vi "Send PCP command.vi"(0 "PSU type":T1, 1 "PCP":T2, 7 "SP":dbl, 11 "error out 2":errorcluster) -> (6 "d(0.0)":dbl, 8 "Final motor voltage update made":bool, 10 "Updated motor voltage pending":bool, 15 "error out":errorcluster)   [LabVIEW 2011]
uses:
  High Level/PCP High Level Commands.ctl
  PSU Type.ctl
  PCP Commands.ctl
  PCP Command definer.ctl
  Magna Interface/Magna Commands.ctl
  Magna Interface/Magna Command Definer.ctl
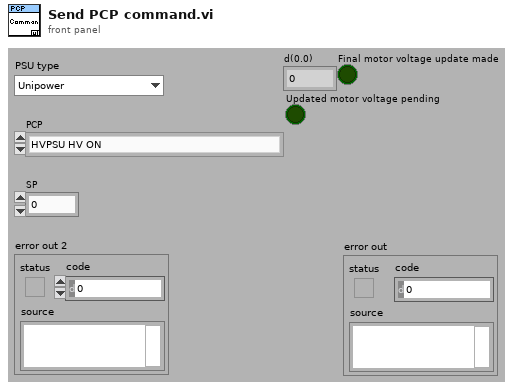
[diagram p1: front panel]
types:
  T1 = typedef "PSU Type.ctl" = enum16{"Unipower", "Magna 8.3A", "Magna 12A", "None"}
  T2 = typedef "PCP High Level Commands.ctl" = enum16{"HVPSU HV ON", "HVPSU HV OFF", "PCP PC", "PCP Local", "Update Motor Voltage", "Update Cable Resistance", "Final Motor Voltage", "Final Resistance"}
  T3 = typedef "PCP Commands.ctl" = enum16{"do not use HE - Help", "RDd - Most used inputs", "RA - All analog inputs", "RE n Reset DO n", "SE n Set DO n", "RP - Get digital inputs", "VA d Set AO A  Motor Volt", "VB d Set AO B  Cable Resistance", "VEr - Get Version", "DYp - Depth counter", "DR - Reset Depth Counter", "DS n Set Depth options(0-3)", "do not use ME - Manual mode enabled", "MD - Manual mode disabled", "ID - Get ID(2001)", "TS - Get Timestamp", "TO d(s)  Set timeout", "do not use LO n Start Loop Mode(1,2)", "AL n RD&LO variation", "ST - Stop Loop Mode"}
  T4 = typedef "PCP Command definer.ctl" = cluster{"Action":T3, "n(0)":i32, "d(0.0)":dbl}
  T5 = typedef "Magna Commands.ctl" = enum16{"Read Inputs", "HV ON", "HV OFF", "Set Resistance", "Set Head Voltage SP"}
  T6 = typedef "Magna Command Definer.ctl" = cluster{"Action":T5, "n(0)":i32, "d(0.0)":dbl}
  T7 = typedef "Options  All pages and custom.ctl" = cluster{"P 1 (App)":T8, "P 2":T9, "P 3":T10, "P 4":T12, "P 5":T17, "P 6 (Err)":T18, "P 7 (Expert)":T19, "P 8 (Depth)":T21, "C 1":T22, "C 2":T23}
  T8 = typedef "Options Page 1 (App).ctl" = cluster{"Result files":path, "PCP Interface":string, "Tractor/Stroker Interface":string, "Tractor Interface":string, "Modem Status Interface":string, "Audible Alarm":bool, "Force alarm on Technical":bool, "Force alarm on HH":bool, "Force alarm on LL":bool, "Force alarm on H":bool, "Force alarm on L":bool}
  T9 = typedef "Options Page 2.ctl" = cluster{"Solenoid & Relay latching time":u16, "Tractor relay 1":dbl, "Tractor relay 2":dbl, "Tractor Solenoid limit":dbl}
  T10 = typedef "Options Page 3.ctl" = cluster{"Min resistance":dbl, "Max resistance":dbl, "Head voltage range":T11, "Max voltage jump":dbl, "Maximum resistance change":dbl, "Start Telemetry Voltage":dbl, "Start Telemetry Timeout":dbl, "Start Motor Voltage":dbl, "Stop Motor Voltage":dbl, "Pass Mode Warning Voltage":dbl, "Relay Switch Voltage":dbl, "Relay Status Loss Voltage":dbl, "Samples to average":i32, "PSU type DO NOT USE":T1, "Magna OVP":dbl, "Magna Current Limit":dbl}
  T11 = typedef "PCP type List.ctl" = enum16{"0 - 350V", "0 - 450V", "0 - 600V"}
  T12 = typedef "Options Page 4.ctl" = cluster{"Solenoid & Relay latching time":u16, "Stroker relay 1":dbl, "Stroker Relay 2":dbl, "Stroker Solenoid limit":dbl, "Force det.":T13, "Stroke force lim.":dbl, "Anchor Enabled Pressure":dbl, "Tacometer puls":dbl, "Default anchor behavior":T14, "Default stroker behavior":T15, "Default stroker force limit (tonne)":dbl, "Slips Size":T16}
  T13 = typedef "Stroke force selector.ctl" = enum16{"Stroke in = node 1", "Strok out = node 1"}
  T14 = typedef "Default anchor behavior.ctl" = enum16{"Do nothing", "Set Anchor", "Release Anchor"}
  T15 = typedef "Default stroker behavior.ctl" = enum16{"Do nothing", "Stop", "Go Out", "Go In"}
  T16 = typedef "Slips Type Radio.ctl" = enum32{"No Selection", "338 MRS", "3,9 MRS"}
  T17 = typedef "Options Page 5.ctl" = cluster{"Solenoid & Relay latching time":u16, "Driller relay 1":dbl, "Driller Relay 2":dbl, "Driller  Solenoid limit":dbl}
  T18 = typedef "Options Page 6 (Err).ctl" = cluster{"Error and event files":path}
  T19 = typedef "Options Page 7 (Expert).ctl" = cluster{"Show Debug":bool, "Log debug messages":bool, "Additional debug messages":bool, "Start Beagle with Simulator data":bool, "Workshop mode":bool, "Modem baud":u16, "enumCANCOM":bool, "Modem sim":T20, "Telemetry Timeout Disable":i32, "Buffer size":i32, "Upd regular data":bool, "Cable comp":cluster{"VMOD1 Voltage(V)":dbl, "VMOD2 Voltage(V)":dbl}}
  T20 = typedef "Modem simulation setup.ctl" = cluster{"Modem dealay sim":bool, "Sim baud Tx":u16, "Bit Error fraction Tx":dbl, "Sim baud Rx":u16, "Bit Error fraction Rx":dbl}
  T21 = typedef "Options Page 8 (Depth).ctl" = cluster{"Winch Spool Circumference":dbl, "Winch Pulses per Revolution":dbl, "Current Depth":dbl}
  T22 = typedef "Options Custom 1.ctl" = cluster{"Depth Updated":bool, "Depth Offset":dbl}
  T23 = typedef "Options Custom 2.ctl" = cluster{"Placeholder":bool}
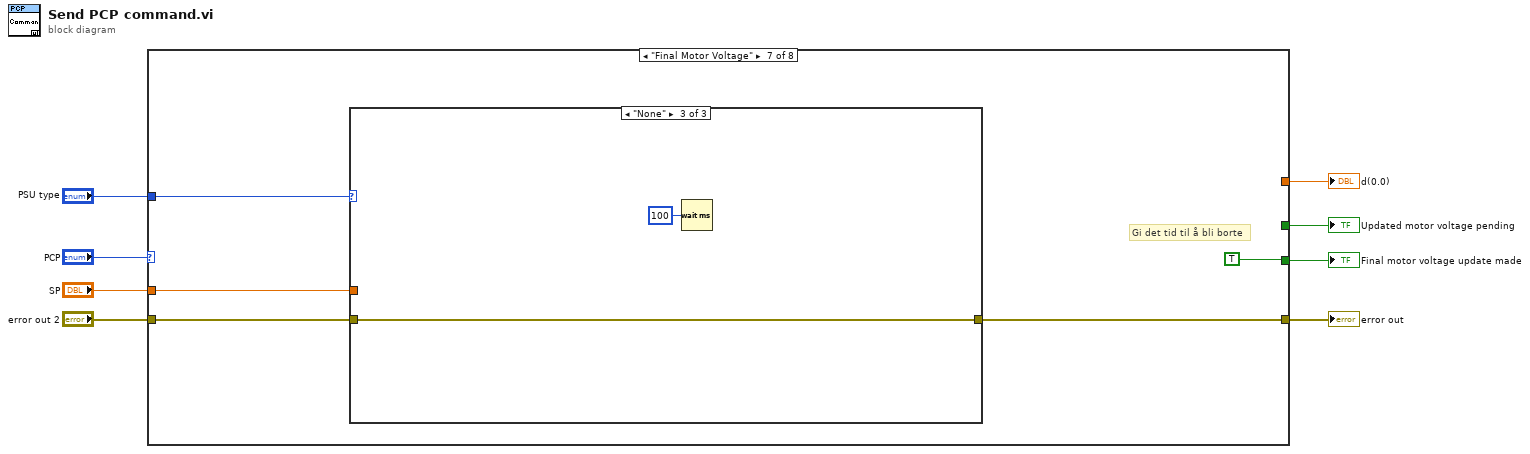
[diagram p0: block diagram]
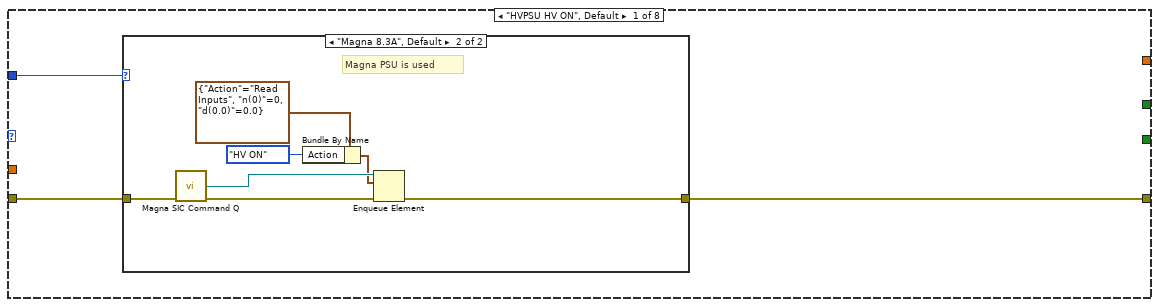
[diagram p2: hidden frame]
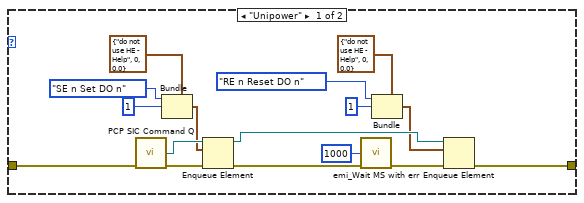
[diagram p3: hidden frame]
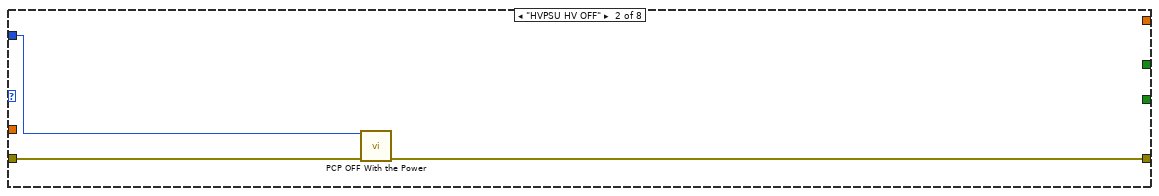
[diagram p4: hidden frame]
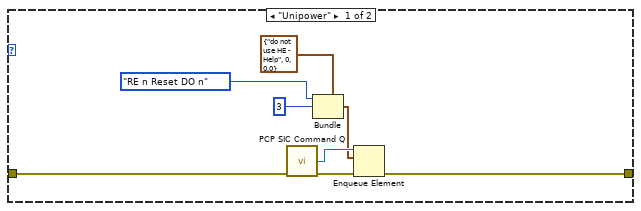
[diagram p6: hidden frame]
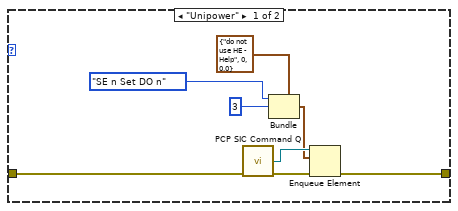
[diagram p8: hidden frame]
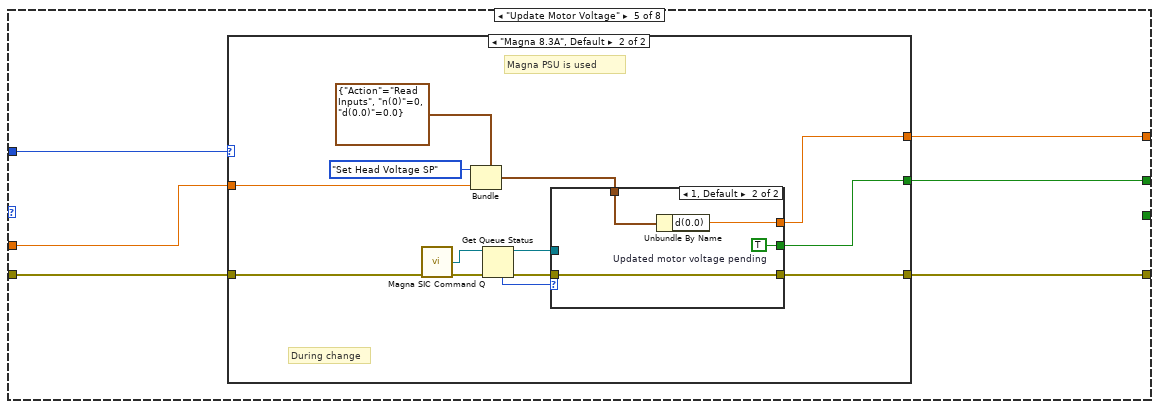
[diagram p9: hidden frame]
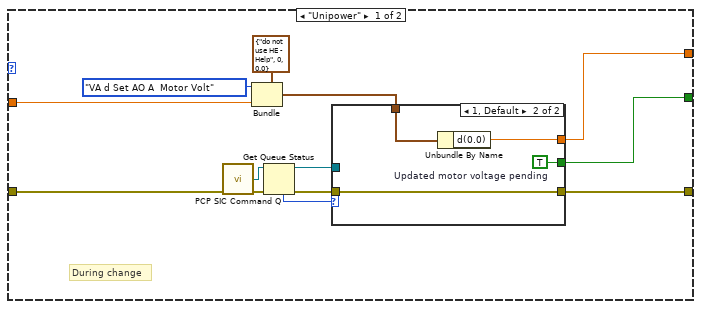
[diagram p10: hidden frame]
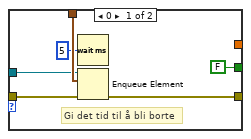
[diagram p11: hidden frame]
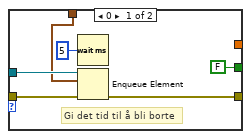
[diagram p12: hidden frame]
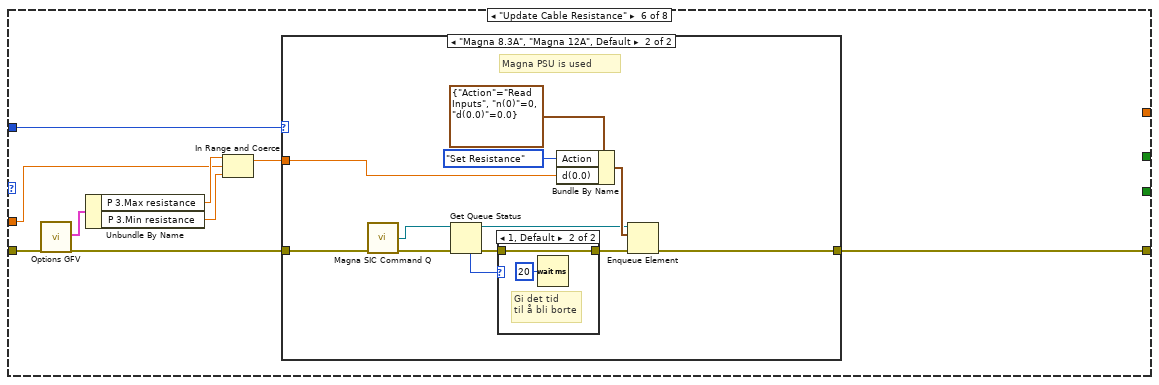
[diagram p13: hidden frame]
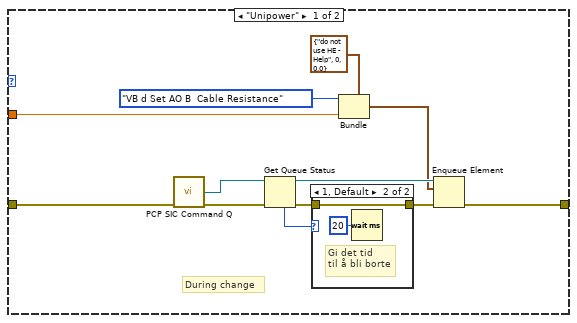
[diagram p14: hidden frame]
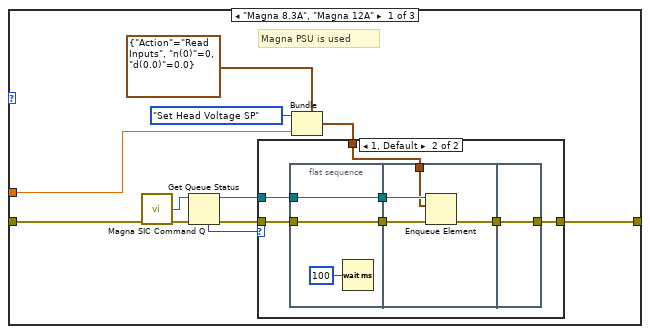
[diagram p17: hidden frame]
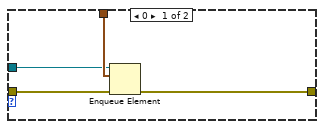
[diagram p18: hidden frame]
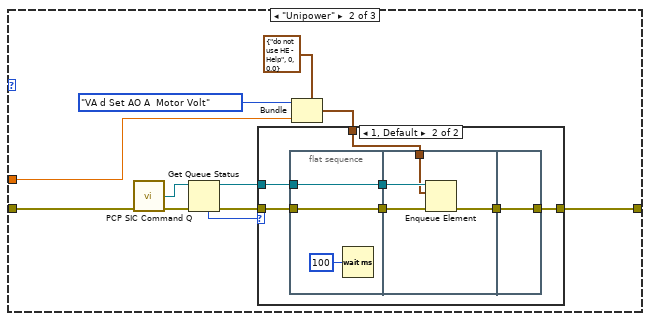
[diagram p19: hidden frame]
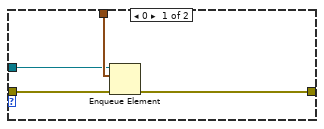
[diagram p20: hidden frame]
diagram:
  n1 = case shown="\"Final Motor Voltage\"" "PCP" {
    tunnel: "error out 2" -> [w11 w36 w40 w52 w67 w119 w157 w226]
    tunnel: "SP" -> [_ _ _ _ w66 w118 w156 w222]
    tunnel: [w10 w37 w39 w51 w65 w115 w155 w228] -> w8
    tunnel: [_ _ _ _ w64 _ _ _] -> w4
    tunnel: [_ _ _ _ w63 _ _ _] -> w3
    tunnel: [_ _ _ _ _ _ TRUE _] -> w2
    tunnel: "PSU type" -> [w9 w35 w38 w50 w62 w114 w153 w220]
    frame "HVPSU HV ON", Default {
      n2 = case shown="\"Magna 8.3A\", Default" w9 {
        tunnel: w11 -> [w13 w34]
        tunnel: [w12 w28] -> w10
        frame "Unipower" {
          n3 = call "PCP SIC Command Q.vi"("error in (no error)"=w13) -> ("PCP cmd Q"=w26:refnum<queue>, "error out"=w27:errorcluster)  [unwired: 13 in]
          n4 = Bundle(cluster=T4 {"Action"=enum."do not use HE - Help", "n(0)"=0, "d(0.0)"=0.0} ("PCP command definer"), "Action"=PCP_Commands."SE n Set DO n", "n(0)"=1) -> (w20:T4)  [unwired: 1 in]
          n5 = Enqueue Element(queue=w26, element=w20, error in (no error)=w27) -> (queue out=w22:refnum<queue>, error out=w25:errorcluster)  [unwired: 1 in, 1 out]
          n6 = call "emi_Wait MS with err.vi"("milliseconds to wait(0)"=u32 1000, "error in (no error)"=w25) -> ("error out"=w23:errorcluster)  [unwired: 13 in]
          n7 = Bundle(cluster=T4 {"Action"=enum."do not use HE - Help", "n(0)"=0, "d(0.0)"=0.0} ("PCP command definer"), "Action"=PCP_Commands."RE n Reset DO n", "n(0)"=1) -> (w18:T4)  [unwired: 1 in]
          n8 = Enqueue Element(queue=w22, element=w18, error in (no error)=w23) -> (error out=w12:errorcluster)  [unwired: 1 in, 2 out]
        }
        frame "Magna 8.3A", Default {
          # "Magna PSU is used"
          n9 = call "Magna SIC Command Q.vi"("error in (no error)"=w34) -> ("queue out"=w32:refnum<queue>, "error out"=w33:errorcluster)  [unwired: 13 in]
          n10 = Bundle By Name(cluster=T6 {"Action"=enum."Read Inputs", "n(0)"=0, "d(0.0)"=0.0} ("element"), "Action"=Magna_Commands."HV ON") -> (w30:T6)
          n11 = Enqueue Element(queue=w32, element=w30, error in (no error)=w33) -> (error out=w28:errorcluster)  [unwired: 1 in, 2 out]
        }
      }
    }
    frame "HVPSU HV OFF" {
      n12 = call "PCP OFF With the Power.vi"("PSU type"=w35, "error In"=w36) -> ("error out"=w37:errorcluster)  [unwired: 13 in]
    }
    frame "PCP PC" {
      n13 = case shown="\"Magna 8.3A\", Default" w38 {
        tunnel: w40 -> [w48 w49]
        tunnel: [w41 w49] -> w39
        frame "Unipower" {
          n14 = call "PCP SIC Command Q.vi"("error in (no error)"=w48) -> ("PCP cmd Q"=w46:refnum<queue>, "error out"=w47:errorcluster)  [unwired: 13 in]
          n15 = Bundle(cluster=T4 {"Action"=enum."do not use HE - Help", "n(0)"=0, "d(0.0)"=0.0} ("PCP command definer"), "Action"=PCP_Commands."RE n Reset DO n", "n(0)"=3) -> (w44:T4)  [unwired: 1 in]
          n16 = Enqueue Element(queue=w46, element=w44, error in (no error)=w47) -> (error out=w41:errorcluster)  [unwired: 1 in, 2 out]
        }
        frame "Magna 8.3A", Default {
          # "Command is not supported"
          # "Magna PSU is used"
        }
      }
    }
    frame "PCP Local" {
      n17 = case shown="\"Magna 8.3A\", Default" w50 {
        tunnel: w52 -> [w60 w61]
        tunnel: [w53 w61] -> w51
        frame "Unipower" {
          n18 = call "PCP SIC Command Q.vi"("error in (no error)"=w60) -> ("PCP cmd Q"=w58:refnum<queue>, "error out"=w59:errorcluster)  [unwired: 13 in]
          n19 = Bundle(cluster=T4 {"Action"=enum."do not use HE - Help", "n(0)"=0, "d(0.0)"=0.0} ("PCP command definer"), "Action"=PCP_Commands."SE n Set DO n", "n(0)"=3) -> (w56:T4)  [unwired: 1 in]
          n20 = Enqueue Element(queue=w58, element=w56, error in (no error)=w59) -> (error out=w53:errorcluster)  [unwired: 1 in, 2 out]
        }
        frame "Magna 8.3A", Default {
          # "Command is not supported"
          # "Magna PSU is used"
        }
      }
    }
    frame "Update Motor Voltage" {
      n21 = case shown="\"Magna 8.3A\", Default" w62 {
        tunnel: w67 -> [w77 w95]
        tunnel: w66 -> [w76 w102]
        tunnel: [w71 w99] -> w65
        tunnel: [w69 w97] -> w64
        tunnel: [w68 w96] -> w63
        frame "Unipower" {
          # "During change"
          n22 = call "PCP SIC Command Q.vi"("error in (no error)"=w77) -> ("PCP cmd Q"=w74:refnum<queue>, "error out"=w75:errorcluster)  [unwired: 13 in]
          n23 = Bundle(cluster=T4 {"Action"=enum."do not use HE - Help", "n(0)"=0, "d(0.0)"=0.0} ("PCP command definer"), "Action"=PCP_Commands."VA d Set AO A  Motor Volt", "d(0.0)"=w76) -> (w79:T4)  [unwired: 1 in]
          n24 = Get Queue Status(queue=w74, error in (no error)=w75) -> (queue out=w70:refnum<queue>, error out=w73:errorcluster, # elements in queue=w72:i32)  [unwired: 1 in, 5 out]
          n25 = case shown="1, Default" w72 {
            tunnel: w79 -> [w86 w89]
            tunnel: w73 -> [w85 w90]
            tunnel: [w84 w90] -> w71
            tunnel: w70 -> [w83 _]
            tunnel: [_ w88] -> w69
            tunnel: [FALSE ("Updated motor voltage pending") w87] -> w68
            frame 0 {
              # "Gi det tid til å bli borte"
              n26 = Wait (ms)(milliseconds to wait=u32 5) -> ()  [unwired: 1 out]
              n27 = Enqueue Element(queue=w83, element=w86, error in (no error)=w85) -> (error out=w84:errorcluster)  [unwired: 1 in, 2 out]
            }
            frame 1, Default {
              w87 = TRUE  # Updated motor voltage pending
              n28 = Unbundle By Name(w89) -> ("d(0.0)"=w88:dbl)
            }
          }
        }
        frame "Magna 8.3A", Default {
          # "Magna PSU is used"
          # "During change"
          n29 = call "Magna SIC Command Q.vi"("error in (no error)"=w95) -> ("queue out"=w93:refnum<queue>, "error out"=w94:errorcluster)  [unwired: 13 in]
          n30 = Bundle(cluster=T6 {"Action"=enum."Read Inputs", "n(0)"=0, "d(0.0)"=0.0} ("element"), "Action"=Magna_Commands."Set Head Voltage SP", "d(0.0)"=w102) -> (w103:T6)  [unwired: 1 in]
          n31 = Get Queue Status(queue=w93, error in (no error)=w94) -> (queue out=w98:refnum<queue>, error out=w101:errorcluster, # elements in queue=w100:i32)  [unwired: 1 in, 5 out]
          n32 = case shown="1, Default" w100 {
            tunnel: w103 -> [w104 w112]
            tunnel: w101 -> [w109 w113]
            tunnel: [w108 w113] -> w99
            tunnel: w98 -> [w107 _]
            tunnel: [_ w111] -> w97
            tunnel: [FALSE ("Updated motor voltage pending") w110] -> w96
            frame 0 {
              # "Gi det tid til å bli borte"
              n33 = Wait (ms)(milliseconds to wait=u32 5) -> ()  [unwired: 1 out]
              n34 = Enqueue Element(queue=w107, element=w104, error in (no error)=w109) -> (error out=w108:errorcluster)  [unwired: 1 in, 2 out]
            }
            frame 1, Default {
              w110 = TRUE  # Updated motor voltage pending
              n35 = Unbundle By Name(w112) -> ("d(0.0)"=w111:dbl)
            }
          }
        }
      }
    }
    frame "Update Cable Resistance" {
      n36 = call "Options GFV.vi"("error in (no error)"=w119) -> ("Options"=w122:T7, "error out"=w116:errorcluster)  [unwired: 16 in, 1 out]
      n37 = Unbundle By Name(w122) -> ("P 3.Max resistance"=w121:dbl, "P 3.Min resistance"=w120:dbl)
      n38 = In Range and Coerce(upper limit=w121, x=w118, lower limit=w120) -> (coerced(x)=w117:dbl)  [unwired: 1 out]
      n39 = case shown="\"Magna 8.3A\", \"Magna 12A\", Default" w114 {
        tunnel: w117 -> [w132 w138]
        tunnel: w116 -> [w125 w146]
        tunnel: [w124 w145] -> w115
        frame "Unipower" {
          # "During change"
          n40 = call "PCP SIC Command Q.vi"("error in (no error)"=w125) -> ("PCP cmd Q"=w126:refnum<queue>, "error out"=w127:errorcluster)  [unwired: 13 in]
          n41 = Get Queue Status(queue=w126, error in (no error)=w127) -> (queue out=w128:refnum<queue>, error out=w131:errorcluster, # elements in queue=w130:i32)  [unwired: 1 in, 5 out]
          n42 = case shown="1, Default" w130 {
            tunnel: w131 -> [w135 w136]
            tunnel: [w135 w136] -> w129
            frame 0 {
            }
            frame 1, Default {
              # "Gi det tid \ntil å bli borte"
              n43 = Wait (ms)(milliseconds to wait=u32 20) -> ()  [unwired: 1 out]
            }
          }
          n44 = Bundle(cluster=T4 {"Action"=enum."do not use HE - Help", "n(0)"=0, "d(0.0)"=0.0} ("PCP command definer"), "Action"=PCP_Commands."VB d Set AO B  Cable Resistance", "d(0.0)"=w132) -> (w123:T4)  [unwired: 1 in]
          n45 = Enqueue Element(queue=w128, element=w123, error in (no error)=w129) -> (error out=w124:errorcluster)  [unwired: 1 in, 2 out]
        }
        frame "Magna 8.3A", "Magna 12A", Default {
          # "Magna PSU is used"
          n46 = call "Magna SIC Command Q.vi"("error in (no error)"=w146) -> ("queue out"=w141:refnum<queue>, "error out"=w142:errorcluster)  [unwired: 13 in]
          n47 = Get Queue Status(queue=w141, error in (no error)=w142) -> (queue out=w140:refnum<queue>, error out=w144:errorcluster, # elements in queue=w143:i32)  [unwired: 1 in, 5 out]
          n48 = case shown="1, Default" w143 {
            tunnel: w144 -> [w150 w151]
            tunnel: [w150 w151] -> w139
            frame 0 {
            }
            frame 1, Default {
              # "Gi det tid \ntil å bli borte"
              n49 = Wait (ms)(milliseconds to wait=u32 20) -> ()  [unwired: 1 out]
            }
          }
          n50 = Bundle By Name(cluster=T6 {"Action"=enum."Read Inputs", "n(0)"=0, "d(0.0)"=0.0} ("element"), "Action"=Magna_Commands."Set Resistance", "d(0.0)"=w138) -> (w148:T6)
          n51 = Enqueue Element(queue=w140, element=w148, error in (no error)=w139) -> (error out=w145:errorcluster)  [unwired: 1 in, 2 out]
        }
      }
    }
    frame "Final Motor Voltage" {
      # "Gi det tid til å bli borte"
      n52 = case shown="\"None\"" w153 {
        tunnel: w157 -> [w160 w195 w218]
        tunnel: w156 -> [w167 w194 _]
        tunnel: [w164 w189 w218] -> w155
        frame "Magna 8.3A", "Magna 12A" {
          # "Magna PSU is used"
          n53 = call "Magna SIC Command Q.vi"("error in (no error)"=w160) -> ("queue out"=w158:refnum<queue>, "error out"=w159:errorcluster)  [unwired: 13 in]
          n54 = Get Queue Status(queue=w158, error in (no error)=w159) -> (queue out=w163:refnum<queue>, error out=w166:errorcluster, # elements in queue=w165:i32)  [unwired: 1 in, 5 out]
          n55 = Bundle(cluster=T6 {"Action"=enum."Read Inputs", "n(0)"=0, "d(0.0)"=0.0} ("element"), "Action"=Magna_Commands."Set Head Voltage SP", "d(0.0)"=w167) -> (w168:T6)  [unwired: 1 in]
          n56 = case shown="1, Default" w165 {
            tunnel: w168 -> [w172 w176]
            tunnel: w166 -> [w171 w179]
            tunnel: [w170 w174] -> w164
            tunnel: w163 -> [w169 w177]
            frame 0 {
              n57 = Enqueue Element(queue=w169, element=w172, error in (no error)=w171) -> (error out=w170:errorcluster)  [unwired: 1 in, 2 out]
            }
            frame 1, Default {
              n58 = flat-sequence {
                tunnel: w179 -> [w180]
                tunnel: [w181] -> w178
                tunnel: w177 -> [w181]
                tunnel: [w180] -> w175
                tunnel: w178 -> [w186]
                tunnel: w176 -> [w185]
                tunnel: w175 -> [w184]
                tunnel: [w183] -> w173
                tunnel: [w187] -> w174
                tunnel: w173 -> [w187]
                frame #0 {
                  n59 = Wait (ms)(milliseconds to wait=u32 100) -> ()  [unwired: 1 out]
                }
                frame #1 {
                  n60 = Enqueue Element(queue=w186, element=w185, error in (no error)=w184) -> (error out=w183:errorcluster)  [unwired: 1 in, 2 out]
                }
                frame #2 {
                }
              }
            }
          }
        }
        frame "Unipower" {
          n61 = call "PCP SIC Command Q.vi"("error in (no error)"=w195) -> ("PCP cmd Q"=w192:refnum<queue>, "error out"=w193:errorcluster)  [unwired: 13 in]
          n62 = Get Queue Status(queue=w192, error in (no error)=w193) -> (queue out=w188:refnum<queue>, error out=w191:errorcluster, # elements in queue=w190:i32)  [unwired: 1 in, 5 out]
          n63 = Bundle(cluster=T4 {"Action"=enum."do not use HE - Help", "n(0)"=0, "d(0.0)"=0.0} ("PCP command definer"), "Action"=PCP_Commands."VA d Set AO A  Motor Volt", "d(0.0)"=w194) -> (w197:T4)  [unwired: 1 in]
          n64 = case shown="1, Default" w190 {
            tunnel: w197 -> [w202 w206]
            tunnel: w191 -> [w201 w209]
            tunnel: [w200 w204] -> w189
            tunnel: w188 -> [w199 w207]
            frame 0 {
              n65 = Enqueue Element(queue=w199, element=w202, error in (no error)=w201) -> (error out=w200:errorcluster)  [unwired: 1 in, 2 out]
            }
            frame 1, Default {
              n66 = flat-sequence {
                tunnel: w209 -> [w210]
                tunnel: [w211] -> w208
                tunnel: w207 -> [w211]
                tunnel: [w210] -> w205
                tunnel: w208 -> [w216]
                tunnel: w206 -> [w215]
                tunnel: w205 -> [w214]
                tunnel: [w213] -> w203
                tunnel: [w217] -> w204
                tunnel: w203 -> [w217]
                frame #0 {
                  n67 = Wait (ms)(milliseconds to wait=u32 100) -> ()  [unwired: 1 out]
                }
                frame #1 {
                  n68 = Enqueue Element(queue=w216, element=w215, error in (no error)=w214) -> (error out=w213:errorcluster)  [unwired: 1 in, 2 out]
                }
                frame #2 {
                }
              }
            }
          }
        }
        frame "None" {
          n69 = Wait (ms)(milliseconds to wait=u32 100) -> ()  [unwired: 1 out]
        }
      }
    }
    frame "Final Resistance" {
      n70 = call "Options GFV.vi"("error in (no error)"=w226) -> ("Options"=w227:T7, "error out"=w225:errorcluster)  [unwired: 16 in, 1 out]
      n71 = Unbundle By Name(w227) -> ("P 3.Max resistance"=w224:dbl, "P 3.Min resistance"=w223:dbl)
      n72 = In Range and Coerce(upper limit=w224, x=w222, lower limit=w223) -> (coerced(x)=w221:dbl)  [unwired: 1 out]
      n73 = case shown="\"Magna 8.3A\", Default" w220 {
        tunnel: [w229 w244] -> w228
        tunnel: w225 -> [w238 w250]
        tunnel: w221 -> [w237 w253]
        frame "Unipower" {
          n74 = call "PCP SIC Command Q.vi"("error in (no error)"=w238) -> ("PCP cmd Q"=w231:refnum<queue>, "error out"=w232:errorcluster)  [unwired: 13 in]
          n75 = Get Queue Status(queue=w231, error in (no error)=w232) -> (queue out=w233:refnum<queue>, error out=w236:errorcluster, # elements in queue=w235:i32)  [unwired: 1 in, 5 out]
          n76 = case shown="1, Default" w235 {
            tunnel: w236 -> [w241 w242]
            tunnel: [w241 w242] -> w234
            frame 0 {
            }
            frame 1, Default {
              # "Gi det tid \ntil å bli borte"
              n77 = Wait (ms)(milliseconds to wait=u32 100) -> ()  [unwired: 1 out]
            }
          }
          n78 = Bundle(cluster=T4 {"Action"=enum."do not use HE - Help", "n(0)"=0, "d(0.0)"=0.0} ("PCP command definer"), "Action"=PCP_Commands."VB d Set AO B  Cable Resistance", "d(0.0)"=w237) -> (w230:T4)  [unwired: 1 in]
          n79 = Enqueue Element(queue=w233, element=w230, error in (no error)=w234) -> (error out=w229:errorcluster)  [unwired: 1 in, 2 out]
        }
        frame "Magna 8.3A", Default {
          # "Magna PSU is used"
          n80 = call "Magna SIC Command Q.vi"("error in (no error)"=w250) -> ("queue out"=w251:refnum<queue>, "error out"=w252:errorcluster)  [unwired: 13 in]
          n81 = Get Queue Status(queue=w251, error in (no error)=w252) -> (queue out=w245:refnum<queue>, error out=w255:errorcluster, # elements in queue=w254:i32)  [unwired: 1 in, 5 out]
          n82 = case shown="1, Default" w254 {
            tunnel: w255 -> [w256 w257]
            tunnel: [w256 w257] -> w247
            frame 0 {
            }
            frame 1, Default {
              # "Gi det tid \ntil å bli borte"
              n83 = Wait (ms)(milliseconds to wait=u32 100) -> ()  [unwired: 1 out]
            }
          }
          n84 = Bundle(cluster=T6 {"Action"=enum."Read Inputs", "n(0)"=0, "d(0.0)"=0.0} ("element"), "Action"=Magna_Commands."Set Resistance", "d(0.0)"=w253) -> (w246:T6)  [unwired: 1 in]
          n85 = Enqueue Element(queue=w245, element=w246, error in (no error)=w247) -> (error out=w244:errorcluster)  [unwired: 1 in, 2 out]
        }
      }
    }
  }
  "error out" <- w8
  "d(0.0)" <- w4
  "Updated motor voltage pending" <- w3
  "Final motor voltage update made" <- w2
